vi "Set Main FPGA Chassis Slots Programming Mode.vi"(8 "error in (no error)":errorcluster, 10 "serverName in":string="10.0.18.244", 11 "Item Ref in":T1 format="%.0x") -> (0 "error out":errorcluster, 2 "serverName out":string="10.0.18.244", 3 "Item Ref out":T1 format="%.0x")   [LabVIEW 2016, in "Scan Engine Custom Device.lvlib"]
doc: "Goal of this VI is to set the slot \"Programming Mode\" property for recent cRIO chassis (NI-904x, NI-905x,...) in accordance to control \"FPGA / Scan interface mode\" control of Target main Configuration page, in \"Othe Settings\" section.\n------------------------------------------------------------------------------------------------------\nIMPLEMENTATION\nThis VI checks the value of property \"FPGA / Scan interface mode\" of Target Configuration Page."
uses:
  Scan Engine Custom Device.lvlib
  <vilib>/NI Veristand/Custom Device Tools/Custom Device Utility Library/Custom Device Utility Library.lvlib
  <vilib>/NI Veristand/Custom Device Offline API/Custom Device Offline API.lvlib
  NationalInstruments.VeriStand.SystemDefinitionAPI
  Type Defs/FPGAScanInterfaceMode.ctl
  <vilib>/NI Veristand/Custom Device API/Custom Device Item Ref.ctl
  <vilib>/NI Veristand/Custom Device API/Custom Device API.lvlib
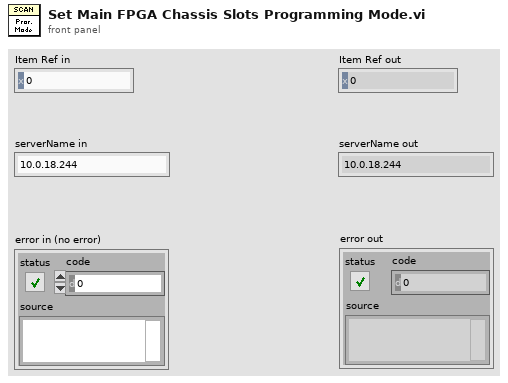
[diagram p1: front panel]
types:
  T1 = typedef "Custom Device API.lvlib/Custom Device Item Ref.ctl" = u64
  T2 = typedef "Scan Engine Custom Device.lvlib/FPGAScanInterfaceMode.ctl" = enum16{"Use Current", "FPGA", "Scan mode"}
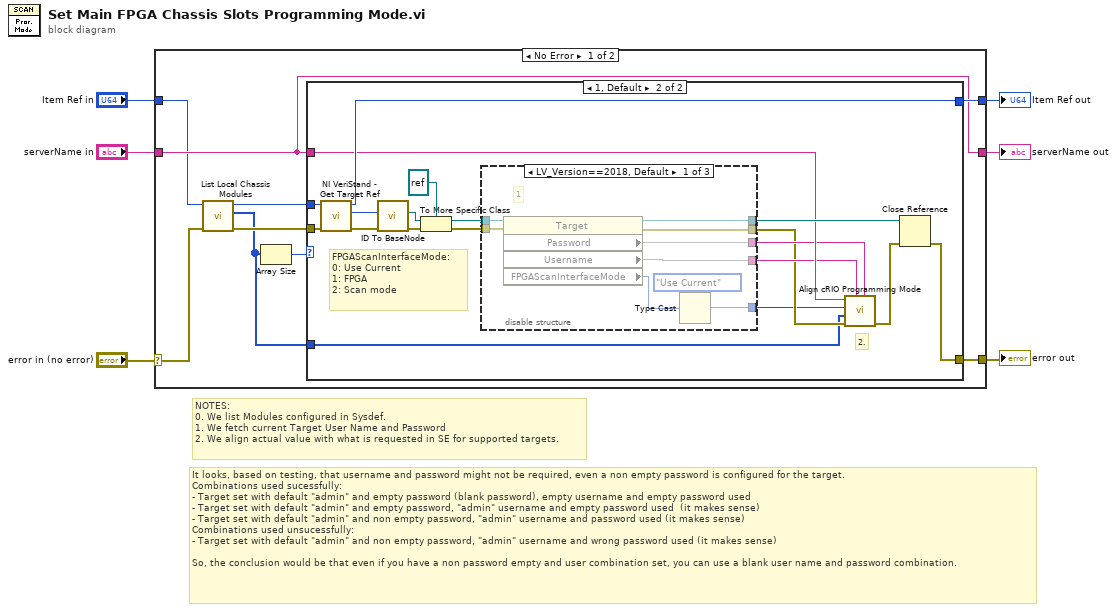
[diagram p0: block diagram]
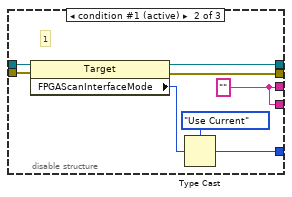
[diagram p3: hidden frame]
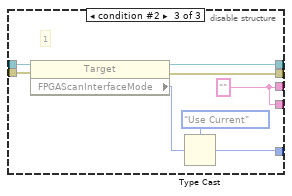
[diagram p4: hidden frame]
diagram:
  # "It looks, based on testing, that username and password might not be required, even a non empty password is configured for the target.\nCombinations used sucessfully:\n- Target set with default \"admin\" and empty password (blank password), empty username and empty password used\n- Target set with default \"admin\" and empty password, \"admin\" username and empty password used  (it makes sense)\n- Target set with default \"admin\" and non empty password, \"admin\" username and password used (it makes sense)\nCombinations used unsucessfully:\n- Target set with default \"admin\" and non empty password, \"admin\" username and wrong password used (it makes sense)\n\nSo, the conclusion would be that even if you have a non password empty and user combination set, you can use a blank user name and password combination."
  # "NOTES:\n0. We list Modules configured in Sysdef.\n1. We fetch current Target User Name and Password\n2. We align actual value with what is requested in SE for supported targets."
  n1 = case shown="No Error" "error in (no error)" {
    selector: "error in (no error)" -> [w11 w64]
    tunnel: [w14 w64] -> w5
    tunnel: "Item Ref in" -> [w12 w63]
    tunnel: [w15 w63] -> w3
    tunnel: "serverName in" -> [w13 w62]
    tunnel: [w13 w62] -> w1
    frame No Error {
      n2 = call "List Local Chassis Modules.vi"("error in (no error)"=w11, "Item Ref in"=w12) -> ("error out"=w9:errorcluster, "Local Slots #"=w7:u32[], "Item Ref out"=w10:T1)  [unwired: 7 in]
      n3 = Array Size(array=w7) -> (size(s)=w8:i32)
      n4 = case shown="1, Default" w8 {
        tunnel: [w17 w32] -> w15
        tunnel: [w16 w28] -> w14
        tunnel: w13 -> [_ w25]
        tunnel: w10 -> [w17 w20]
        tunnel: w9 -> [w16 w19]
        tunnel: w7 -> [_ w18]
        frame 0 {
          # "No modules configured in Local Chassis in Sysdef."
        }
        frame 1, Default {
          # "2."
          # "FPGAScanInterfaceMode:\n0: Use Current\n1: FPGA\n2: Scan mode"
          n5 = call <vilib>:"NI VeriStand - Get Target Ref.vi"("error in"=w19, "Item Ref in"=w20) -> ("error out"=w31:errorcluster, "Target Ref"=w36:T1, "Item Ref out"=w32:T1)  [unwired: 6 in, 1 out]
          n6 = call <vilib>:"ID To BaseNode.vi"("error in (no error)"=w31, "ID in"=w36) -> ("error out"=w30:errorcluster, "BaseNode"=w34:refnum<k24>)  [unwired: 7 in, 1 out]
          n7 = To More Specific Class(target class=refnum<k24> refnum, reference=w34, error in=w30) -> (specific class reference=w35:refnum<k24>, error out=w29:errorcluster)
          n8 = disable-structure shown="LV_Version==2018, Default" {
            disable-tunnel: w35 -> [w45 w53 w61]
            disable-tunnel: w29 -> [w44 w52 w60]
            disable-tunnel: [w43 w51 w59] -> w27
            disable-tunnel: [w42 w48 w57] -> w24
            disable-tunnel: [w41 w48 w57] -> w23
            disable-tunnel: [w40 w50 w58] -> w22
            disable-tunnel: [w37 w47 w54] -> w21
            frame condition #0 {
              # "1"
              n9 = property class="Target"(reference=w45, error in=w44) -> (reference out=w43:refnum<k24>, error out=w40:errorcluster, "Password"=w42, "Username"=w41, "FPGAScanInterfaceMode"=w39:u16)
              n10 = Type Cast(type=FPGAScanInterfaceMode."Use Current" ("Enum"), x=w39) -> (*(type *) &x=w37:T2)
            }
            frame condition #1 (active) {
              w48 = ""
              # "1"
              n11 = property class="Target"(reference=w53, error in=w52) -> (reference out=w51:refnum<k24>, error out=w50:errorcluster, "FPGAScanInterfaceMode"=w49:u16)
              n12 = Type Cast(type=FPGAScanInterfaceMode."Use Current" ("Enum"), x=w49) -> (*(type *) &x=w47:T2)
            }
            frame condition #2 {
              w57 = ""
              # "1"
              n13 = property class="Target"(reference=w61, error in=w60) -> (reference out=w59:refnum<k24>, error out=w58:errorcluster, "FPGAScanInterfaceMode"=w56:u16)
              n14 = Type Cast(type=FPGAScanInterfaceMode."Use Current" ("Enum"), x=w56) -> (*(type *) &x=w54:T2)
            }
          }
          n15 = call "Align cRIO Programming Mode.vi"("Password"=w24, "User Name"=w23, "error in (no error)"=w22, "Local Slots #"=w18, "FPGAScanInterfaceMode"=w21, "Target (localhost)"=w25) -> ("error out"=w26:errorcluster)  [unwired: 3 in, 2 out]
          n16 = Close Reference(reference=w27, error in (no error)=w26) -> (error out=w28:errorcluster)
        }
      }
    }
    frame Error {
    }
  }
  "error out" <- w5
  "Item Ref out" <- w3
  "serverName out" <- w1
